vi "serial_nanovna_handler.vi"(9 "button_get_trace_data":bool, 10 "button_serial_connect":bool, 11 "scan_command_get":string) -> (0 "error out":errorcluster, 4 "new_data_available":bool, 6 "read_buffer_out":string)   [LabVIEW 2025]
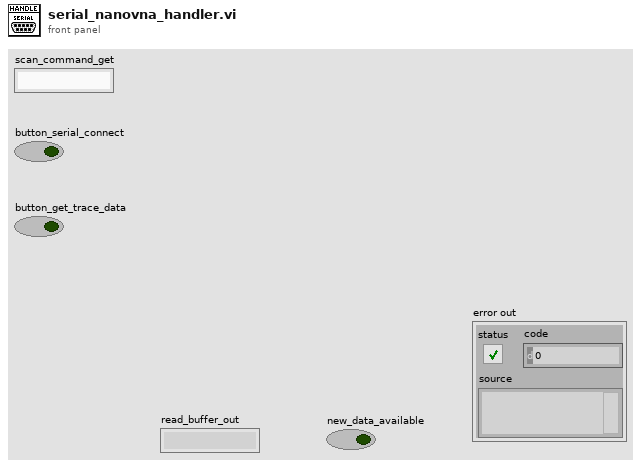
[diagram p1: front panel]
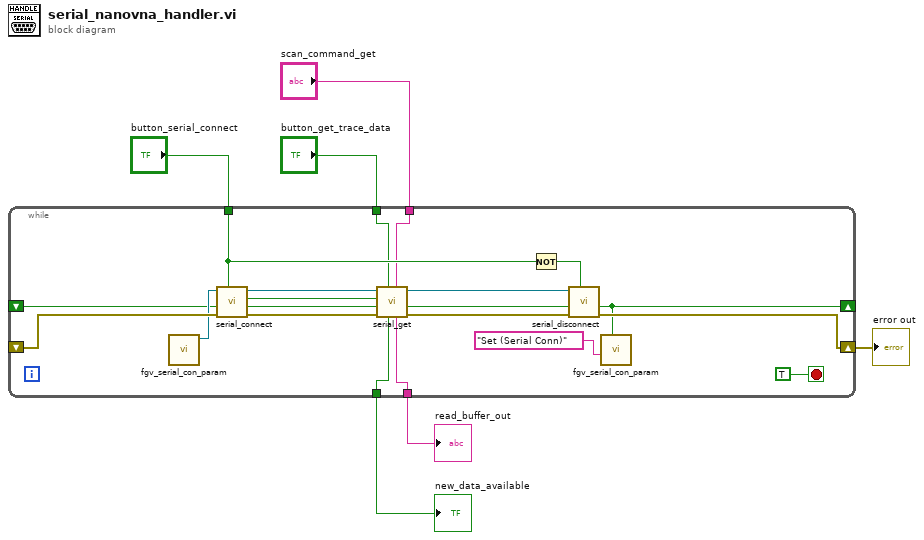
[diagram p0: block diagram]
diagram:
  n1 = while {
    tunnel: "button_serial_connect" -> [w18]
    shift-right: [w15] -> w5
    shift-left: _ -> [w16]
    tunnel: "button_get_trace_data" -> [w12]
    tunnel: "scan_command_get" -> [w11]
    shift-right: [w9] -> _
    shift-left: _ -> [w10]
    tunnel: [w8] -> w2
    tunnel: [w7] -> w1
    stop <- TRUE stop-if-true
    n2 = call "fgv_serial_con_param.vi"() -> ("serial_port_get"=w13:refnum<visa-resource-name>)  [unwired: 7 in, 4 out]
    n3 = call "serial_connect.vi"("button_serial_connect"=w18, "error_in"=w16, "serial_connected_in"=w10, "VISA_resource"=w13) -> ("error out"=w25:errorcluster, "serial_connected_out"=w26:bool, "new_connection"=w22:bool, "VISA_refnum_out"=w20:refnum<visa-resource-name>)  [unwired: 4 in]
    n4 = call "serial_get.vi"("command"=w11, "serial_send"=w12, "error in (no error)"=w25, "serial_connected_in"=w26, "new_connection"=w22, "VISA_refnum_in"=w20) -> ("error out"=w24:errorcluster, "serial_connected_out"=w21:bool, "VISA_Refnum_out"=w19:refnum<visa-resource-name>, "read_buffer_out"=w7:string, "new_data_available"=w8:bool)  [unwired: 1 in]
    n5 = Not(x=w18) -> (.not. x?=w23:bool)
    n6 = call "serial_disconnect.vi"("serial_disconnect"=w23, "error in"=w24, "serial_connected in"=w21, "VISA Refnum in"=w19) -> ("error out"=w15:errorcluster, "serial_connected_out"=w9:bool)  [unwired: 6 in]
    n7 = call "fgv_serial_con_param.vi"("serial_conn_set"=w9, "mode"="Set (Serial Conn)") -> ()  [unwired: 5 in, 5 out]
  }
  "new_data_available" <- w2
  "error out" <- w5
  "read_buffer_out" <- w1
